vi "Get DDG Lite Pulses Per Exposure.vi"(10 "ui32Pulses":u32, 11 "channel":u32(ring)=65535 items=["AT_DDGLite_ChannelA"=1073741824, "AT_DDGLite_ChannelB"=1073741825, "AT_DDGLite_ChannelC"=1073741826]) -> (2 "ui32Pulses out":u32, 3 "function return":u32)   [LabVIEW 2018, in "AndorSDK.lvlib"]
doc: "EXPNETTYPE unsigned int WINAPI GetDDGLitePulsesPerExposure(AT_DDGLiteChannelId channel, at_u32 * ui32Pulses);"
uses:
  AndorSDK.lvlib
  ATMCD32D.dll
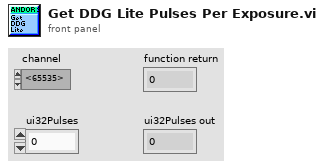
[diagram p1: front panel]
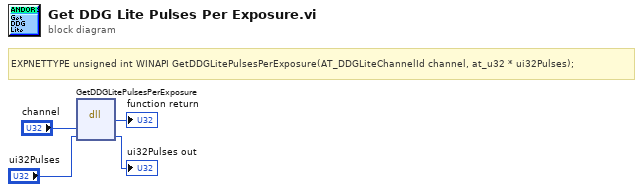
[diagram p0: block diagram]
diagram:
  # "EXPNETTYPE unsigned int WINAPI GetDDGLitePulsesPerExposure(AT_DDGLiteChannelId channel, at_u32 * ui32Pulses);"
  n1 = dll-call lib="PTH2babs E\nPersönliches02 - Arbeit03-HiwijobsLabviewCodelibANDOR\tAndor SDK\nATMCD32D.*" fn="GetDDGLitePulsesPerExposure"("channel"="channel", "ui32Pulses"="ui32Pulses") -> (→"function return":u32, "ui32Pulses"=→"ui32Pulses out":u32)  [unwired: 4 in, 2 out]
